vi "Read Count Measurement (Mask Test).vi"(8 "error in (no error)":errorcluster, 11 "VISA resource name":refnum<visa-resource-name>) -> (0 "error out":errorcluster, 1 "Acquired Waveform Count":dbl, 2 "Elapsed Time (s)":dbl, 3 "VISA resource name out":refnum<visa-resource-name>, 5 "Failed Waveform Count":dbl)   [LabVIEW 2015, in "Agilent 2000 3000 X-Series.lvlib"]
doc: "Returns the measurement of mask test."
uses:
  <instrlib>/Agilent 2000 3000 X-Series/Agilent 2000 3000 X-Series.lvlib
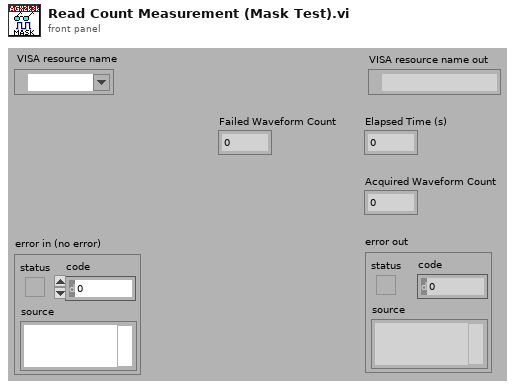
[diagram p1: front panel]
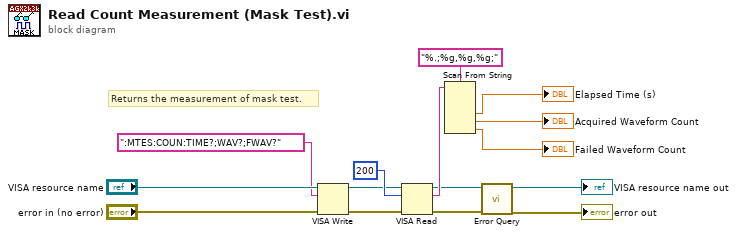
[diagram p0: block diagram]
diagram:
  # "Returns the measurement of mask test."
  n1 = VISA Write(VISA resource name="VISA resource name", write buffer=":MTES:COUN:TIME?;WAV?;FWAV?", error in (no error)="error in (no error)") -> (VISA resource name out=w5:refnum<visa-resource-name>, error out=w7:errorcluster)  [unwired: 1 out]
  n2 = VISA Read(VISA resource name=w5, byte count=u32 200, error in (no error)=w7) -> (VISA resource name out=w4:refnum<visa-resource-name>, read buffer=w10:string, error out=w6:errorcluster)  [unwired: 1 out]
  n3 = Scan From String(format string="%.;%g,%g,%g;", input string=w10) -> (output 1=→"Elapsed Time (s)":dbl, output 2=→"Acquired Waveform Count":dbl, output 3=→"Failed Waveform Count":dbl)  [unwired: 2 in, 6 out]
  n4 = call <instrlib>:"Error Query.vi"("error in (no error)"=w6, "VISA resource name"=w4) -> ("error out"=→"error out":errorcluster, "VISA resource name out"=→"VISA resource name out":refnum<visa-resource-name>)  [unwired: 8 out]
